vi "GetOneQueueStatus.vi"(8 "error in":errorcluster, 10 "priority":i32, 11 "queues in":refnum<class "CLM_PriorityLocalMessage.lvclass">) -> (0 "error out":errorcluster, 1 "max queue size":i32, 2 "# elements in queue":i32, 3 "queues out":refnum<class "CLM_PriorityLocalMessage.lvclass">, 4 "# pending remove":i32, 5 "priority out":i32, 6 "# pending insert":i32)   [LabVIEW 2013, in "CLM_PriorityLocalMessage.lvclass"]
uses:
  CLM_PriorityLocalMessage.lvclass
  CLM_PriorityLocalMessage.lvclass/CLM_PriorityLocalMessage.ctl
  LocalMessage_Queue/CLM_LocalMessage_Queue.lvclass/CLM_LocalMessage_Queue.ctl
  LocalMessage_Queue/CLM_LocalMessage_Queue.lvclass
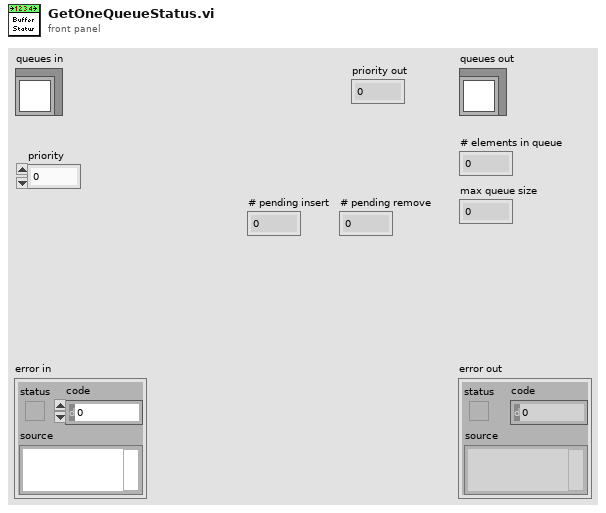
[diagram p1: front panel]
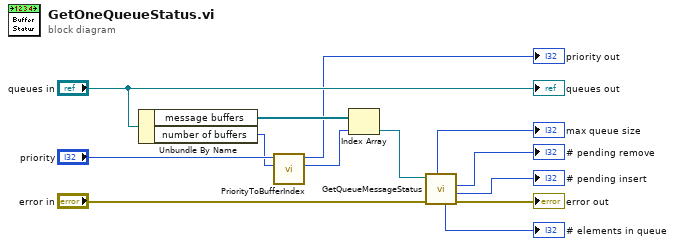
[diagram p0: block diagram]
diagram:
  n1 = Unbundle By Name("queues in") -> ("message buffers"=w4:refnum<class "CLM_LocalMessage_Queue.lvclass">[], "number of buffers"=w5:i32)
  n2 = call "PriorityToBufferIndex.vi"("number of buffers"=w5, "priority"="priority") -> ("buffer index"=w3:i32, "priority out"=→"priority out":i32)  [unwired: 6 in, 2 out]
  n3 = Index Array(array=w4, index=w3) -> (element=w2:refnum<class "CLM_LocalMessage_Queue.lvclass">)
  n4 = call "GetQueueMessageStatus.vi"("error in"="error in", "message ref in"=w2) -> ("error out"=→"error out":errorcluster, "# pending insert"=→"# pending insert":i32, "# pending remove"=→"# pending remove":i32, "# elements in queue"=→"# elements in queue":i32, "max queue size"=→"max queue size":i32)  [unwired: 2 in, 3 out]
  "queues out" <- "queues in"
